vi "_Destroy.vi"(8 "error in (no error)":errorcluster, 11 "Wavelength Meter in":refnum<class "Wavelength Meter.lvclass">) -> (0 "error out":errorcluster)   [LabVIEW 2009, in "Wavelength Meter.lvclass"]
uses:
  Wavelength Meter.lvclass
  Utility Classes/Readable/Readable.lvclass
  HighFinesse WS5/HighFinesse WS5.lvlib
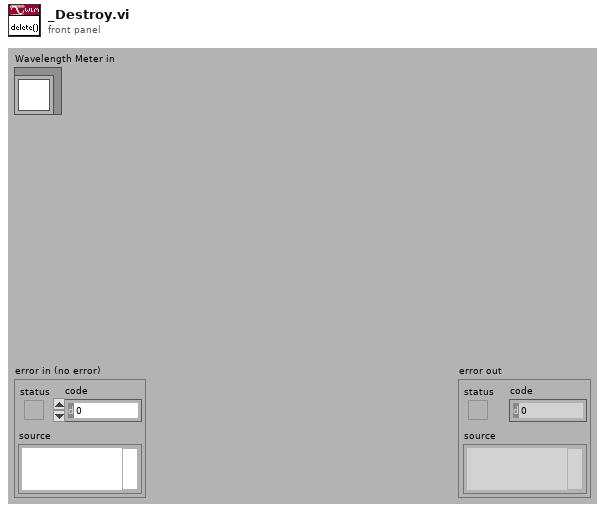
[diagram p1: front panel]
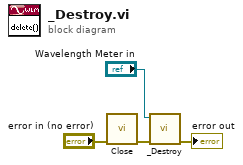
[diagram p0: block diagram]
diagram:
  n1 = call "Close.vi"("error in (no error)"="error in (no error)") -> ("error out"=w1:errorcluster)  [unwired: 1 in, 9 out]
  n2 = call-parent "_Destroy.vi"("error in (no error)"=w1, "Instrument in"="Wavelength Meter in") -> ("error out"=→"error out":errorcluster)  [unwired: 9 out]
